vi "GetType.vi"(8 "error in (no error)":errorcluster, 11 "Set Output Line Msg":refnum<class "Set Output Line Msg.lvclass">) -> (0 "error out":errorcluster, 2 "Data Sample":variant, 3 "Set Output Line Msg":refnum<class "Set Output Line Msg.lvclass">)   [LabVIEW 2021, in "BNT_ULx.lvlib" / "Set Output Line Msg.lvclass"]
uses:
  Set Output Line Msg.lvclass
  Set Output Line Msg.lvclass/Set Output Line Msg.ctl
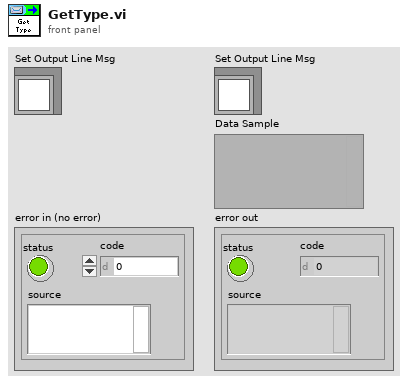
[diagram p1: front panel]
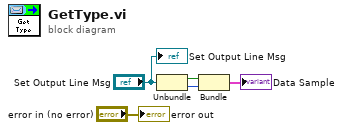
[diagram p0: block diagram]
diagram:
  n1 = Unbundle("Set Output Line Msg") -> (w2:bool, w1:i32)
  n2 = Bundle("Value"=w2, "Line"=w1) -> (→"Data Sample":cluster{"Value":bool, "Line":i32})  [unwired: 1 in]
  "error out" <- "error in (no error)"
  "Set Output Line Msg" <- "Set Output Line Msg"
